vi "5.4.vi"() -> ()   [LabVIEW 2022 SP3]
panel:
  in  "Frequency 2":dbl=10.1 format="%#_13g"
  in  "Frequency":dbl=10.1 format="%#_13g"
  out "XY Graph 2":cluster{"Y":dbl[], "Y":dbl[]}[](graph)
  in  "Amplitude 2":dbl=1.0 caption="Amplitude"
  in  "Phase 2":dbl format="%#_13g"
  in  "Phase":dbl format="%#_13g"
  in  "Amplitude":dbl=1.0
  # "Aditya Singh\n    2315005"
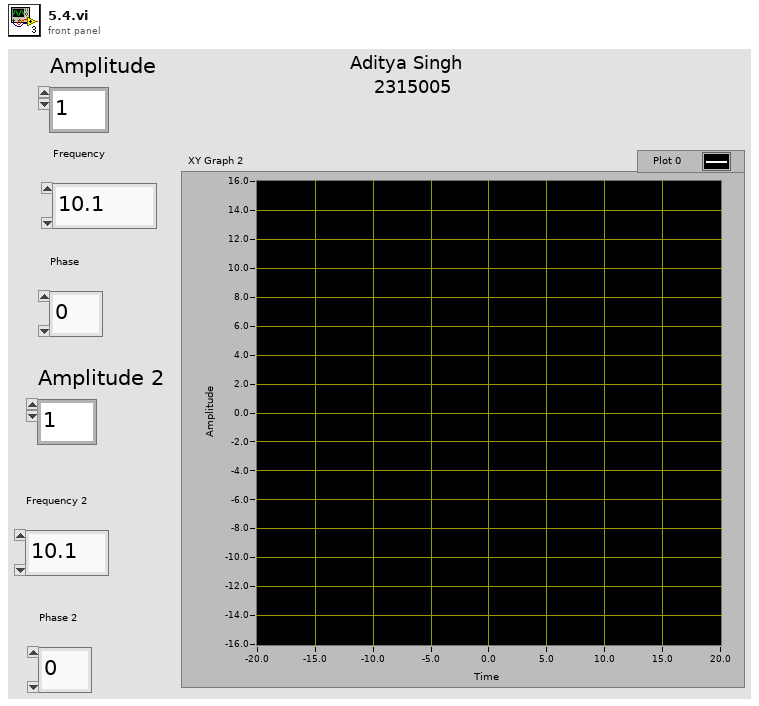
[diagram p1: front panel]
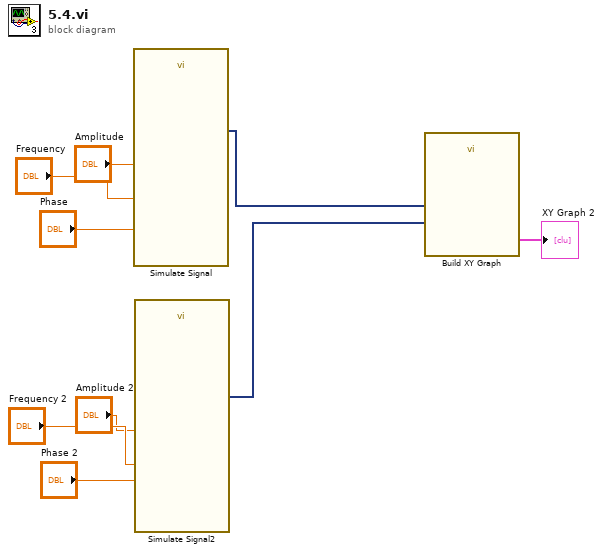
[diagram p0: block diagram]
diagram:
  n1 = call "Simulate Signal"("Frequency"="Frequency", "Amplitude"="Amplitude", "Phase"="Phase") -> ("Sine"=w2:dynamicdata)  [unwired: 11 in, 1 out]
  n2 = call "Simulate Signal2"("Frequency"="Frequency 2", "Amplitude"="Amplitude 2", "Phase"="Phase 2") -> ("Sine"=w1:dynamicdata)  [unwired: 11 in, 1 out]
  n3 = call "Build XY Graph"("Y Input"=w1, "X Input"=w2) -> ("XY Graph"=→"XY Graph 2":cluster{"X":dbl[], "Y":dbl[]}[])  [unwired: 8 in, 1 out]
